vi "SLL DE Compare DO Channel Enum and MAX Channel.vi"(8 "error in (no error)":errorcluster, 11 "Digital Output Channels":refnum<k21>[](array[refnum])) -> (0 "error out":errorcluster, 3 "Channels Out":refnum<k21>[](array[refnum]), 5 "Pass?":bool)   [LabVIEW 2009]
doc: "This VI will check and seperate all Analog Inputs listed in enum form global Channel list\n\nCreated by Yogesh Redemptor, \nCopyright © 2008, Soliton Technologies.\nAll rights reserved."
uses:
  Controls/SLL DE List of Digital Outputs.ctl
panel:
  in  "List of Digital Outputs":T1=enum."STATION1_STOP TEST"
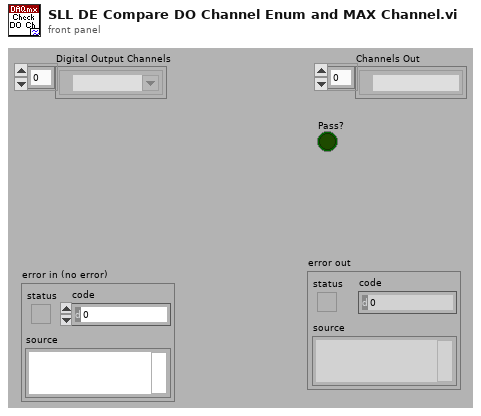
[diagram p1: front panel]
types:
  T1 = typedef "SLL DE List of Digital Outputs.ctl" = enum16{"STATION1_START TEST", "STATION1_STOP TEST", "STATION1_LIGHT1", "STATION1_LIGHT2", "STATION1_LIGHT3", "STATION2_START TEST", "STATION2_STOP TEST", "STATION2_LIGHT1", "STATION2_LIGHT2", "STATION2_LIGHT3", "STATION3_START TEST", "STATION3_STOP TEST", "STATION3_LIGHT1", "STATION3_LIGHT2", "STATION3_LIGHT3", "STATION4_START TEST", "STATION4_STOP TEST", "STATION4_LIGHT1", "STATION4_LIGHT2", "STATION4_LIGHT3"}
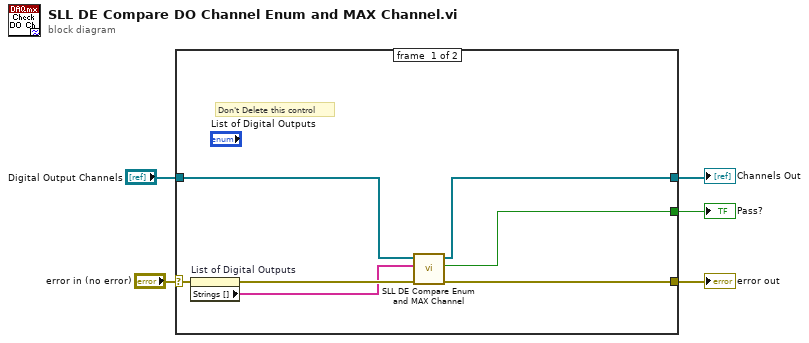
[diagram p0: block diagram]
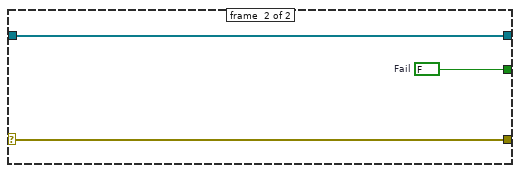
[diagram p2: hidden frame]
diagram:
  n1 = case shown="No Error" "error in (no error)" {
    selector: "error in (no error)" -> [w12 w15]
    tunnel: [w10 w15] -> w4
    tunnel: "Digital Output Channels" -> [w7 w14]
    tunnel: [w8 w13] -> w2
    tunnel: [w9 w14] -> w1
    frame #0 {
      # "Don't Delete this control"
      n2 = property on="List of Digital Outputs" class="Enum (strict)"(error in=w12) -> (error out=w11:errorcluster, "Strings []"=w6:string[])  [unwired: 1 in, 1 out]
      n3 = call "SLL DE Compare Enum and MAX Channel.vi"("error in (no error)"=w11, "Strings []"=w6, "Channels In"=w7) -> ("error out"=w10:errorcluster, "Pass?"=w8:bool, "Channels Out"=w9:refnum<k21>[])  [unwired: 6 in]
    }
    frame #1 {
      w13 = FALSE  # Fail
    }
  }
  "error out" <- w4
  "Pass?" <- w2
  "Channels Out" <- w1
